vi "LaunchProcess.vi"(11 "SMO Reference":refnum<class "SMO.lvclass">) -> ()   [LabVIEW 2013, in "SMO.lvclass"]
doc: "Launches the Process VIs.\n\n---------------------------------------------------------------\nJKI State Machine Objects™\nhttp://jki.net/state-machine-objects/\nCopyright (C) 2005-2015, JKI <info@jki.net>\nALL RIGHTS RESERVED"
uses:
  SMO.lvclass
panel:
  # "For instructions on how to use the JKI State Machine Objects, examples and video tutorials, visit:\nhttp://jki.net/state-machine-objects/\n\nJKI State Machine Objects™\nhttp://jki.net/state-machine-objects/\nCopyright (C) 2005-2015, JKI <info@jki.net>\nALL RIGHTS RESERVED"
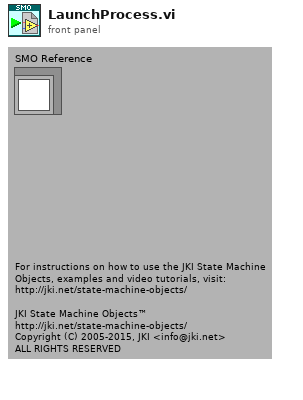
[diagram p1: front panel]
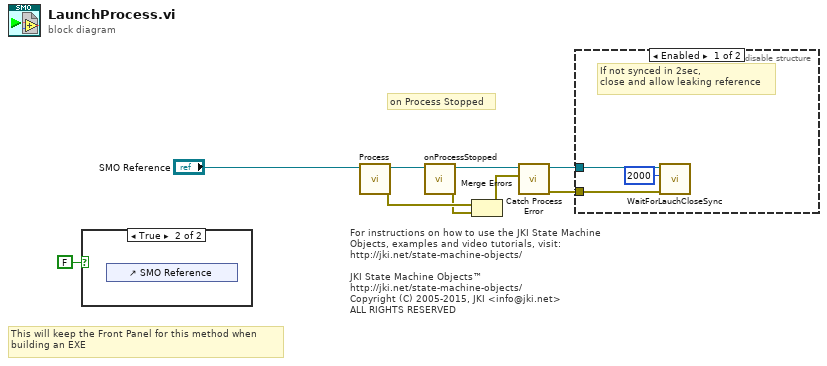
[diagram p0: block diagram]
diagram:
  # "on Process Stopped"
  # "This will keep the Front Panel for this method when\nbuilding an EXE"
  # "For instructions on how to use the JKI State Machine Objects, examples and video tutorials, visit:\nhttp://jki.net/state-machine-objects/\n\nJKI State Machine Objects™\nhttp://jki.net/state-machine-objects/\nCopyright (C) 2005-2015, JKI <info@jki.net>\nALL RIGHTS RESERVED"
  n1 = case shown="True" FALSE {
    frame False {
    }
    frame True {
      n2 = control-ref of="SMO Reference"() -> ()  [unwired: 1 out]
    }
  }
  n3 = call-dynamic "Process.vi"("SMO"="SMO Reference") -> ("error out"=w5:errorcluster, "SMO out"=w7:refnum<class "SMO.lvclass">)  [unwired: 9 in]
  n4 = call-dynamic "onProcessStopped.vi"("SMO"=w7) -> ("error out"=w4:errorcluster, "SMO out"=w6:refnum<class "SMO.lvclass">)  [unwired: 9 in]
  n5 = Merge Errors(w5, w4) -> (w3:errorcluster)
  n6 = call "Catch Process Error.vi"("Process Error"=w3, "SMO"=w6) -> ("error out"=w1:errorcluster, "SMO out"=w2:refnum<class "SMO.lvclass">)  [unwired: 8 in]
  n7 = disable-structure shown="Enabled" {
    disable-tunnel: w2 -> [w12 _]
    disable-tunnel: w1 -> [w10 _]
    frame Enabled {
      # "If not synced in 2sec, \nclose and allow leaking reference"
      n8 = call "WaitForLauchCloseSync.vi"("error in (no error)"=w10, "timeout in ms (-1)"=2000, "SMO"=w12) -> ()  [unwired: 7 in, 2 out]
    }
    frame Disabled {
    }
  }
